vi "Read StandardEvents.vi"(8 "error in (no error)":errorcluster, 11 "JQMHCore in":refnum<class "JQMHModule.lvclass">) -> (0 "error out":errorcluster, 2 "StandardEvents":T1, 3 "JQMHCore out":refnum<class "JQMHModule.lvclass">)   [LabVIEW 2024, in "JQMHModule.lvclass"]
uses:
  JQMHModule.lvclass
  StandardEvents.ctl
  StopEventArgs.ctl
  JQMHModule.lvclass/JQMHModule.ctl
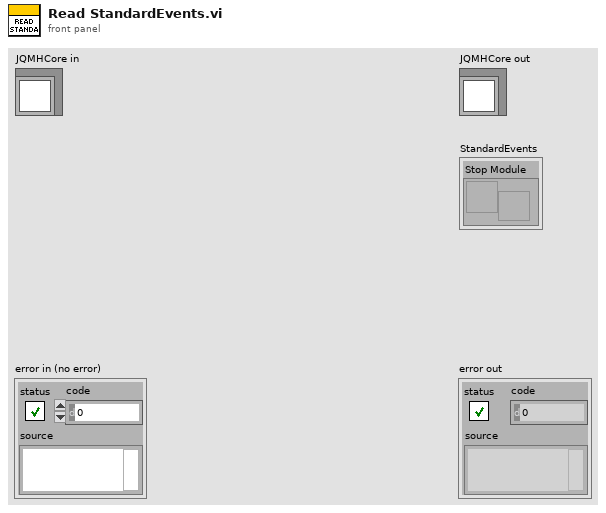
[diagram p1: front panel]
types:
  T1 = typedef "JQMHModule.lvclass/StandardEvents.ctl" = cluster{"Stop Module":refnum<user-event>}
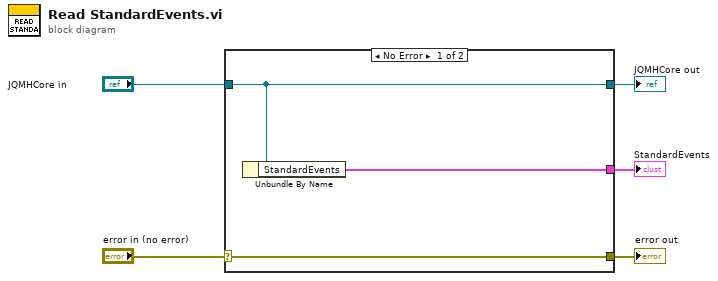
[diagram p0: block diagram]
diagram:
  n1 = case shown="No Error" "error in (no error)" {
    selector: "error in (no error)" -> [w8 w9]
    tunnel: [w8 w9] -> w4
    tunnel: [w7 w10] -> w2
    tunnel: "JQMHCore in" -> [w7 w10]
    tunnel: [w6 _] -> w1
    frame No Error {
      n2 = Unbundle By Name(w7) -> ("StandardEvents"=w6:T1)
    }
    frame Error {
    }
  }
  "error out" <- w4
  "JQMHCore out" <- w2
  "StandardEvents" <- w1
